vi "2022_day10.vi"() -> ()   [LabVIEW 2021]
panel:
  out "Task 2":string
  out "Task 1":i32
  in  "Switch":bool caption="Ex. Data  vs.  User Data"
  # "RUAKHBEK"
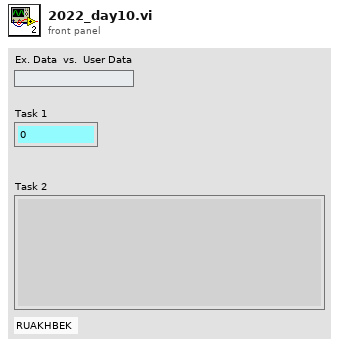
[diagram p1: front panel]
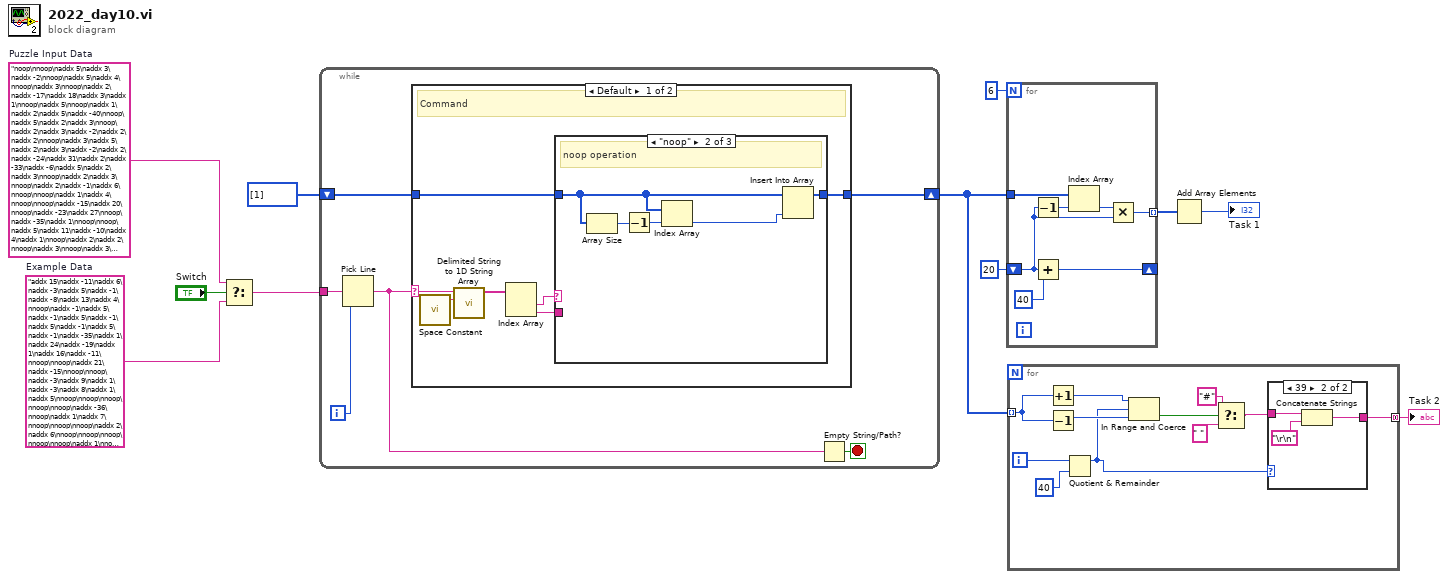
[diagram p0: block diagram]
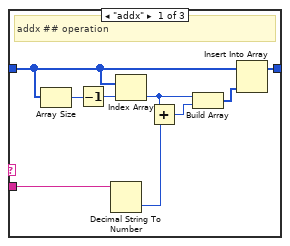
[diagram p2: hidden frame]
diagram:
  w10 = "noop\nnoop\naddx 5\naddx 3\naddx -2\nnoop\naddx 5\naddx 4\nnoop\naddx 3\nnoop\naddx 2\naddx -17\naddx 18\naddx 3\naddx 1\nnoop\naddx 5\nnoop\naddx 1\naddx 2\naddx 5\naddx -40\nnoop\naddx 5\naddx 2\naddx 3\nnoop\naddx 2\naddx 3\naddx -2\naddx 2\naddx 2\nnoop\naddx 3\naddx 5\naddx 2\naddx 3\naddx -2\naddx 2\naddx -24\naddx 31\naddx 2\naddx -33\naddx -6\naddx 5\naddx 2\naddx 3\nnoop\naddx 2\naddx 3\nnoop\naddx 2\naddx -1\naddx 6\nnoop\nnoop\naddx 1\naddx 4\nnoop\nnoop\naddx -15\naddx 20\nnoop\naddx -23\naddx 27\nnoop\naddx -35\naddx 1\nnoop\nnoop\naddx 5\naddx 11\naddx -10\naddx 4\naddx 1\nnoop\naddx 2\naddx 2\nnoop\naddx 3\nnoop\naddx 3\naddx 2\nnoop\naddx 3\naddx 2\naddx 11\naddx -4\naddx 2\naddx -38\naddx -1\naddx 2\nnoop\naddx 3\naddx 5\naddx 2\naddx -7\naddx 8\naddx 2\naddx 2\nnoop\naddx 3\naddx 5\naddx 2\naddx -25\naddx 26\naddx 2\naddx 8\naddx -1\naddx 2\naddx -2\naddx -37\naddx 5\naddx 3\naddx -1\naddx 5\nnoop\naddx 22\naddx -21\naddx 2\naddx 5\naddx 2\naddx 13\naddx -12\naddx 4\nnoop\nnoop\naddx 5\naddx 1\nnoop\nnoop\naddx 2\nnoop\naddx 3\nnoop\nnoop"  # Puzzle Input Data
  w9 = "addx 15\naddx -11\naddx 6\naddx -3\naddx 5\naddx -1\naddx -8\naddx 13\naddx 4\nnoop\naddx -1\naddx 5\naddx -1\naddx 5\naddx -1\naddx 5\naddx -1\naddx 5\naddx -1\naddx -35\naddx 1\naddx 24\naddx -19\naddx 1\naddx 16\naddx -11\nnoop\nnoop\naddx 21\naddx -15\nnoop\nnoop\naddx -3\naddx 9\naddx 1\naddx -3\naddx 8\naddx 1\naddx 5\nnoop\nnoop\nnoop\nnoop\nnoop\naddx -36\nnoop\naddx 1\naddx 7\nnoop\nnoop\nnoop\naddx 2\naddx 6\nnoop\nnoop\nnoop\nnoop\nnoop\naddx 1\nnoop\nnoop\naddx 7\naddx 1\nnoop\naddx -13\naddx 13\naddx 7\nnoop\naddx 1\naddx -33\nnoop\nnoop\nnoop\naddx 2\nnoop\nnoop\nnoop\naddx 8\nnoop\naddx -1\naddx 2\naddx 1\nnoop\naddx 17\naddx -9\naddx 1\naddx 1\naddx -3\naddx 11\nnoop\nnoop\naddx 1\nnoop\naddx 1\nnoop\nnoop\naddx -13\naddx -19\naddx 1\naddx 3\naddx 26\naddx -30\naddx 12\naddx -1\naddx 3\naddx 1\nnoop\nnoop\nnoop\naddx -9\naddx 18\naddx 1\naddx 2\nnoop\nnoop\naddx 9\nnoop\nnoop\nnoop\naddx -1\naddx 2\naddx -37\naddx 1\naddx 3\nnoop\naddx 15\naddx -21\naddx 22\naddx -6\naddx 1\nnoop\naddx 2\naddx 1\nnoop\naddx -10\nnoop\nnoop\naddx 20\naddx 1\naddx 2\naddx 2\naddx -6\naddx -11\nnoop\nnoop\nnoop"  # Example Data
  n1 = Select(t=w10, s="Switch", f=w9) -> (s? t:f=w8:string)
  n2 = while {
    tunnel: w8 -> [w17]
    shift-right: [w12] -> w2
    shift-left: i32[] [1] -> [w14]
    i -> [w13]
    stop <- w16 stop-if-true
    n3 = Pick Line(multi-line string=w17, line index=w13) -> (output string=w15:string)  [unwired: 1 in]
    n4 = case shown="Default" w15 {
      selector: w15 -> [w24 _]
      tunnel: w14 -> [w18 w40]
      tunnel: [w19 w40] -> w12
      frame Default {
        # "Command"
        n5 = call <vilib>:"Space Constant.vi"() -> ("String"=w23:string)
        n6 = call <vilib>:"Delimited String to 1D String Array.vi"("delimiter"=w23, "delimited string"=w24) -> ("string array"=w22:string[])  [unwired: 9 in]
        n7 = Index Array(array=w22) -> (element #1=w21:string, element #2=w20:string)  [unwired: 2 in]
        n8 = case shown="\"noop\"" w21 {
          tunnel: w20 -> [w27 _ _]
          tunnel: [w33 w38 w39] -> w19
          tunnel: w18 -> [w31 w36 w39]
          frame "addx" {
            # "addx ## operation"
            n9 = Array Size(array=w31) -> (size(s)=w32:i32)
            n10 = Decrement(x=w32) -> (x-1=w30:i32)
            n11 = Decimal String To Number(string=w27) -> (number=w28:i32)  [unwired: 2 in, 1 out]
            n12 = Index Array(array=w31, index=w30) -> (element=w26:i32)
            n13 = Add(x=w26, y=w28) -> (x+y=w25:i32)
            n14 = Build Array(w26, w25) -> (w29:i32[])
            n15 = Insert Into Array(array=w31, new element=w29) -> (w33:i32[])  [unwired: 1 in]
          }
          frame "noop" {
            # "noop operation"
            n16 = Array Size(array=w36) -> (size(s)=w37:i32)
            n17 = Decrement(x=w37) -> (x-1=w35:i32)
            n18 = Index Array(array=w36, index=w35) -> (element=w34:i32)
            n19 = Insert Into Array(array=w36, new element=w34) -> (w38:i32[])  [unwired: 1 in]
          }
          frame Default {
          }
        }
      }
      frame "" {
        # "End of file"
      }
    }
    n20 = Empty String/Path?(string/path=w15) -> (empty?=w16:bool)
  }
  n21 = for {
    N: 6 -> [_]
    tunnel: w2 -> [w47]
    shift-right: [w45] -> _
    shift-left: 20 ("Num") -> [w43]
    tunnel: [w42] -> w4 mode=indexing
    n22 = Decrement(x=w43) -> (x-1=w41:i32)
    n23 = Add(x=w43, y=40 ("Num")) -> (x+y=w45:i32)
    n24 = Index Array(array=w47, index=w41) -> (element=w44:i32)
    n25 = Multiply(x=w44, y=w43) -> (x*y=w42:i32)
  }
  n26 = for {
    tunnel: w2 -> [w58] mode=indexing
    tunnel: [w52] -> w1 mode=concatenating
    i -> [w48]
    n27 = Increment(x=w58) -> (x+1=w56:i32)
    n28 = Decrement(x=w58) -> (x-1=w57:i32)
    n29 = Quotient & Remainder(x=w48, y=40) -> (x-y*floor(x/y)=w49:i32)  [unwired: 1 out]
    n30 = In Range and Coerce(upper limit=w56, x=w49, lower limit=w57) -> (In Range?=w53:bool)  [unwired: 1 out]
    n31 = Select(t="#", s=w53, f=" ") -> (s? t:f=w51:string)
    n32 = case shown="39" w49 {
      tunnel: [w59 w61] -> w52
      tunnel: w51 -> [w59 w62]
      frame Default {
      }
      frame 39 {
        n33 = Concatenate Strings(w62, "\r\n") -> (w61:string)
      }
    }
  }
  "Task 2" <- w1
  n34 = Add Array Elements(numeric array=w4) -> (sum=→"Task 1":i32)
